vi "Show One Plot.vi"() -> ()   [LabVIEW 2012]
uses:
  <vilib>/Utility/miscctls.llb/LVRangeTypeDef.ctl
  <vilib>/Utility/miscctls.llb/LVPointDoubleTypeDef.ctl
  Type/_Data Operation.ctl
  <vilib>/printing/EasyPrintingControls.llb/layout_options.ctl
  <vilib>/printing/EasyPrintingControls.llb/orientation.ctl
  <vilib>/printing/EasyPrintingControls.llb/panel_scaling_for_page.ctl
  <vilib>/printing/EasyPrintingControls.llb/margins.ctl
  <vilib>/printing/EasyPrintingControls.llb/margin_values.ctl
  <vilib>/printing/EasyPrintingControls.llb/measurement_system.ctl
  <vilib>/printing/EasyPrintingControls.llb/printer_options.ctl
  <vilib>/printing/EasyPrintingControls.llb/printing_method.ctl
  <vilib>/printing/EasyPrintingControls.llb/color_or_monochrome.ctl
  <vilib>/printing/EasyPrintingControls.llb/page_header_options.ctl
  <vilib>/printing/EasyPrintingControls.llb/page_headers.ctl
  <vilib>/printing/EasyPrintingControls.llb/page_header_content_options.ctl
  <vilib>/printing/EasyPrinting.llb/Easy Print VI Panel or Documentation (path).vi
  <vilib>/Utility/NIReport.llb/NI_ReportGenerationCore.lvlib
panel:
  in  "Data":T3
  in  "Expt#":i32=1 caption="Experiment #"
  out "Scan #":i32=1
  out "Run Time":i32=1 caption="Run Time (ms)"
  out "Plot":cluster{"TIC X":dbl[], "TIC Y":dbl[]}[](graph)
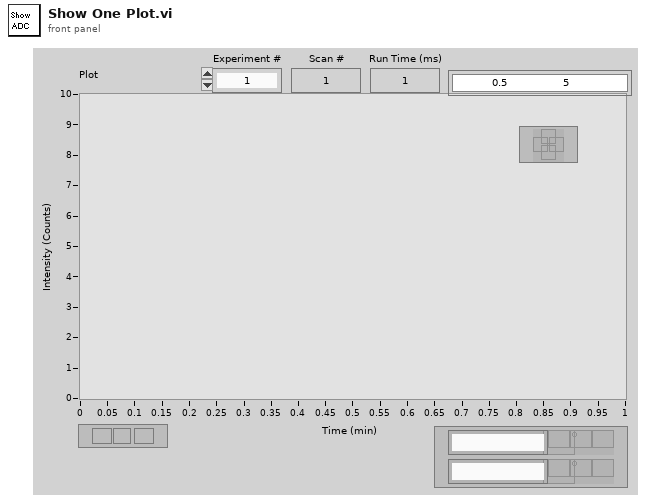
[diagram p1: front panel]
types:
  T1 = typedef "LVRangeTypeDef.ctl" = cluster{"Minimum":dbl, "Maximum":dbl, "Increment":dbl, "Minor Increment":dbl, "Start":dbl}
  T2 = typedef "LVPointDoubleTypeDef.ctl" = cluster{"X":dbl, "Y":dbl}
  T3 = cluster{"YScale.NameLbl.Text":string, "XScale.NameLbl.Text":string, "XScale.Range":T1, "YScale.Range":T1, "Label.Text":string, "Cursor.Cursor Position":T2, "Plot.Bar Plot Style":u8}
  T4 = typedef "_Data Operation.ctl" = enum8{"Initialize", "Get Data", "Set Data", "Close"}
  T5 = typedef "NI_ReportGenerationCore.lvlib/layout_options.ctl" = cluster{"orientation (unchanged)":T6, "panel scaling for page (unchanged)":T7, "margins":T8, "printer options":T11, "page header options":T14}
  T6 = typedef "NI_ReportGenerationCore.lvlib/orientation.ctl" = u16
  T7 = typedef "NI_ReportGenerationCore.lvlib/panel_scaling_for_page.ctl" = u16
  T8 = typedef "NI_ReportGenerationCore.lvlib/margins.ctl" = cluster{"override VI margins (false)":bool, "margins (1.00)":T9, "measurement system (default)":T10}
  T9 = typedef "NI_ReportGenerationCore.lvlib/margin_values.ctl" = cluster{"top":dbl, "left":dbl, "right":dbl, "bottom":dbl}
  T10 = typedef "NI_ReportGenerationCore.lvlib/measurement_system.ctl" = u16
  T11 = typedef "NI_ReportGenerationCore.lvlib/printer_options.ctl" = cluster{"destination printer name (current)":string, "printing method (unchanged)":T12, "color or monochrome (unchanged)":T13}
  T12 = typedef "NI_ReportGenerationCore.lvlib/printing_method.ctl" = u16
  T13 = typedef "NI_ReportGenerationCore.lvlib/color_or_monochrome.ctl" = u16
  T14 = typedef "NI_ReportGenerationCore.lvlib/page_header_options.ctl" = cluster{"page headers (unchanged)":T15, "page header content options":T16}
  T15 = typedef "NI_ReportGenerationCore.lvlib/page_headers.ctl" = u16
  T16 = typedef "NI_ReportGenerationCore.lvlib/page_header_content_options.ctl" = cluster{"Include VI Name":bool, "Include VI Path":bool, "Include Last Modification Date":bool, "Include Date Printed":bool, "Include Page Number":bool, "Include VI Icon":bool}
  T17 = typedef "_Current Data.ctl" = cluster{"Scan#":i32, "Run Time (mS)":i32, "TIC X":dbl[], "TIC Y":dbl[][], "MassRange":cluster{"X Title":string, "X":dbl[], "Y":i32[]}[], "Fixed Mass (amu)":dbl, "Method":T18}
  T18 = typedef "_XML Expt.ctl" = cluster{"StartT(mS)":i32, "#Cycles":i32, "PauseT(uS)":i32, "ScanType":i32, "Polarity":u8, "FixedMass":dbl, "DelayT(mS)":i32, "Active Ch":T19[], "Mass Range":T20[]}
  T19 = typedef "_XML Lens.ctl" = cluster{"Value":dbl, "ChID":u8}
  T20 = typedef "_Mass Range Property.ctl" = cluster{"Start":dbl, "Stop":dbl, "Step Size":dbl, "Steps":i32, "Dwell":dbl, "Parameters":T21[], "Res":T22}
  T21 = typedef "_Mass Range Parameters.ctl" = cluster{"Name":string, "Ch#":u8, "StartV":dbl, "StopV":dbl, "StepV":dbl, "Index":u8}
  T22 = typedef "_RT Res Type.ctl" = u16
  T23 = cluster{"Data":cluster{"X":dbl[], "Y":dbl[]}, "Y Title":string, "X Title":string}
  T24 = typedef "imagedata.ctl" = cluster{"image type":i32, "image depth":i32, "image":u8[], "mask":u8[], "colors":u32[], "Rectangle":cluster{"left":i16, "top":i16, "right":i16, "bottom":i16}}
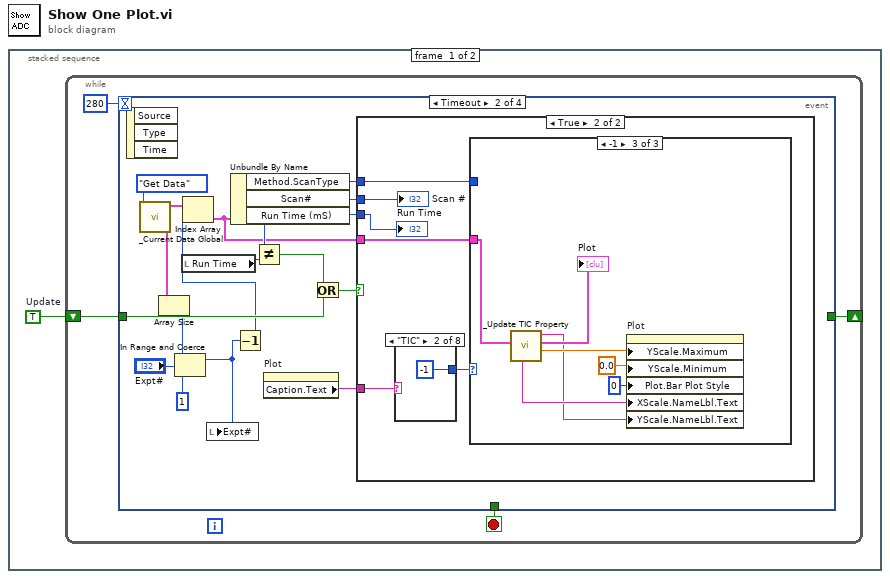
[diagram p0: block diagram]
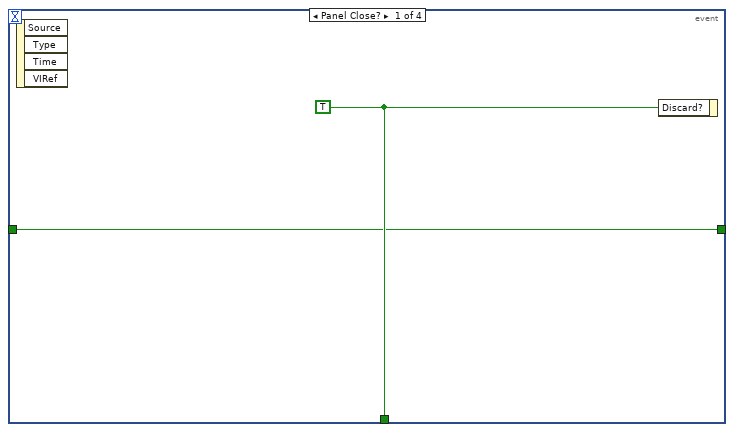
[diagram p2: hidden frame]
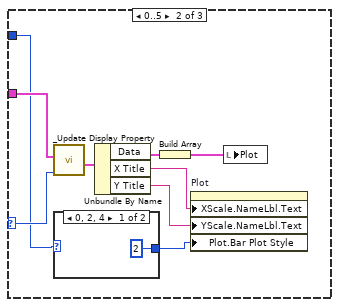
[diagram p5: hidden frame]
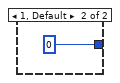
[diagram p6: hidden frame]
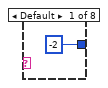
[diagram p7: hidden frame]
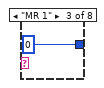
[diagram p8: hidden frame]
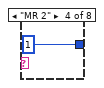
[diagram p9: hidden frame]
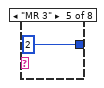
[diagram p10: hidden frame]
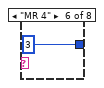
[diagram p11: hidden frame]
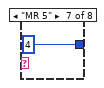
[diagram p12: hidden frame]
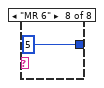
[diagram p13: hidden frame]
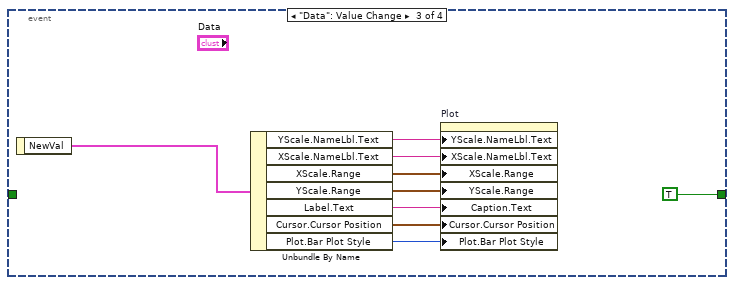
[diagram p14: hidden frame]
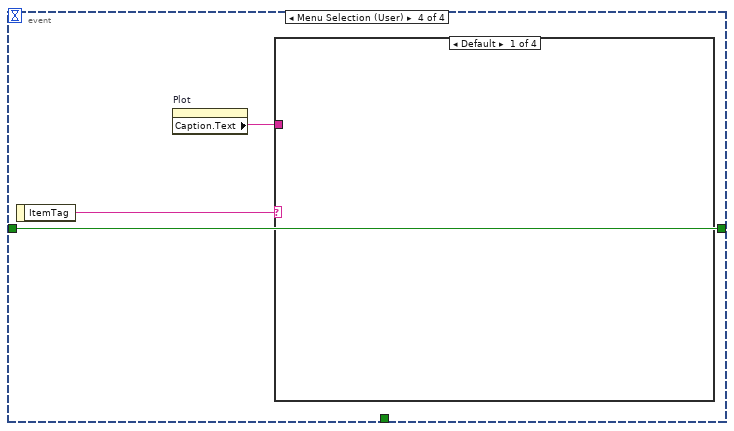
[diagram p15: hidden frame]
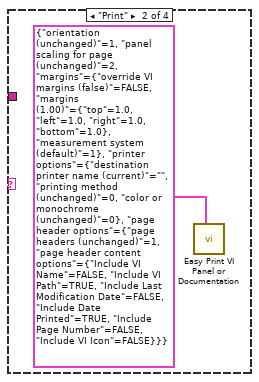
[diagram p16: hidden frame]
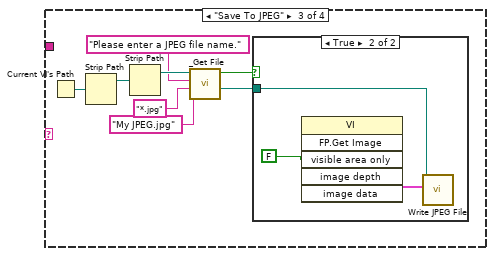
[diagram p17: hidden frame]
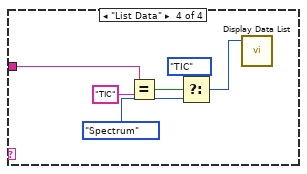
[diagram p19: hidden frame]
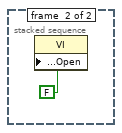
[diagram p20: hidden frame]
diagram:
  n1 = stacked-sequence {
    frame #0 {
      w1 = TRUE  # Update
      n2 = while {
        shift-right: [w2] -> _
        shift-left: w1 -> [w3]
        stop <- w5 stop-if-true
        n3 = event shown="[1] Timeout" {
          selector: _ -> [_ _ _ _]
          dyn-events: _ -> [_ _ _ _]
          timeout: 280 -> [_ _ _ _]
          tunnel: [w7 _ _ _] -> w5
          tunnel: w3 -> [w6 w22 _ w65]
          tunnel: [w6 _ TRUE ("Update") w65] -> w2
          event Panel Close? {
            w7 = TRUE ("Discard?")
            n4 = event-data() -> ()  [unwired: 5 out]
            n5 = event-data("Discard?"=w7) -> ()  [unwired: 1 in, 1 out]
          }
          event Timeout {
            n6 = event-data() -> ()  [unwired: 4 out]
            n7 = call "_Current Data Global.vi"("Operation"=_Data_Operation."Get Data") -> ("CurrentData"=w13:T17[])  [unwired: 3 in, 3 out]
            n8 = Array Size(array=w13) -> (size(s)=w14:i32)
            n9 = In Range and Coerce(upper limit=w14, x="Expt#", lower limit=1) -> (coerced(x)=w10:i32)  [unwired: 1 out]
            n10 = local read "Run Time"() -> (w18:i32)
            n11 = local write "Expt#"(w10) -> ()
            n12 = Decrement(x=w10) -> (x-1=w9:i32)
            n13 = Index Array(array=w13, index=w9) -> (element=w15:T17)
            n14 = Unbundle By Name(w15) -> ("Method.ScanType"=w8:i32, "Scan#"=w19:i32, "Run Time (mS)"=w17:i32)
            n15 = Not Equal?(x=w17, y=w18) -> (x != y?=w16:bool)
            n16 = property on="Plot" class="XYGraph (strict)"() -> ("Caption.Text"=w23:string)  [unwired: 2 in, 2 out]
            n17 = Or(x=w16, y=w22) -> (x .or. y?=w21:bool)
            n18 = case shown="True" w21 {
              tunnel: w23 -> [_ w29]
              tunnel: w17 -> [_ w26]
              tunnel: w19 -> [_ w27]
              tunnel: w15 -> [_ w25]
              tunnel: w8 -> [_ w24]
              frame False {
              }
              frame True {
                n19 = case shown="\"TIC\"" w29 {
                  tunnel: [-2 -1 0 1 2 3 4 5] -> w28
                  frame Default {
                  }
                  frame "TIC" {
                  }
                  frame "MR 1" {
                  }
                  frame "MR 2" {
                  }
                  frame "MR 3" {
                  }
                  frame "MR 4" {
                  }
                  frame "MR 5" {
                  }
                  frame "MR 6" {
                  }
                }
                n20 = case shown="-1" w28 {
                  selector: w28 -> [_ w38 _]
                  tunnel: w25 -> [_ w32 w45]
                  tunnel: w24 -> [_ w31 _]
                  frame Default {
                  }
                  frame 0..5 {
                    n21 = call "_Update Display Property.vi"("MassRange# (0)"=w38, "Current Data"=w32) -> ("Graph Data"=w37:T23)  [unwired: 2 in, 4 out]
                    n22 = case shown="0, 2, 4" w31 {
                      tunnel: [u8 2 ("Plot.Bar Plot Style") u8 0 ("Plot.Bar Plot Style")] -> w30
                      frame 0, 2, 4 {
                      }
                      frame 1, Default {
                      }
                    }
                    n23 = Unbundle By Name(w37) -> ("Data"=w36:cluster{"X":dbl[], "Y":dbl[]}, "X Title"=w34:string, "Y Title"=w33:string)
                    n24 = Build Array(w36) -> (w35:cluster{"X":dbl[], "Y":dbl[]}[])
                    n25 = property on="Plot" class="XYGraph (strict)"("XScale.NameLbl.Text"=w34, "YScale.NameLbl.Text"=w33, "Plot.Bar Plot Style"=w30) -> ()  [unwired: 2 in, 2 out]
                    n26 = local write "Plot"(w35) -> ()
                  }
                  frame -1 {
                    n27 = call "_Update TIC Property.vi"("Current Data"=w45) -> ("YMax"=w43:dbl, "TIC Data"=→"Plot":cluster{"TIC X":dbl[], "Data in cps":dbl[]}[], "YTitle"=w41:string, "XTitle"=w42:string)  [unwired: 7 out]
                    n28 = property on="Plot" class="XYGraph (strict)"("YScale.Maximum"=w43, "YScale.Minimum"=0.0 ("Y Scale.Range:Minimum"), "Plot.Bar Plot Style"=u8 0, "XScale.NameLbl.Text"=w42, "YScale.NameLbl.Text"=w41) -> ()  [unwired: 2 in, 2 out]
                  }
                }
                "Scan #" <- w27
                "Run Time" <- w26
              }
            }
          }
          event "Data": Value Change {
            n29 = event-data() -> ("NewVal"=w63:T3)  [unwired: 1 out]
            n30 = Unbundle By Name(w63) -> ("YScale.NameLbl.Text"=w57:string, "XScale.NameLbl.Text"=w58:string, "XScale.Range"=w59:T1, "YScale.Range"=w60:T1, "Label.Text"=w61:string, "Cursor.Cursor Position"=w62:T2, "Plot.Bar Plot Style"=w56:u8)
            n31 = property on="Plot" class="XYGraph (strict)"("YScale.NameLbl.Text"=w57, "XScale.NameLbl.Text"=w58, "XScale.Range"=w59, "YScale.Range"=w60, "Caption.Text"=w61, "Cursor.Cursor Position"=w62, "Plot.Bar Plot Style"=w56) -> ()  [unwired: 2 in, 2 out]
          }
          event Menu Selection (User) {
            n32 = event-data() -> ("ItemTag"=w67:string)  [unwired: 1 out]
            n33 = property on="Plot" class="XYGraph (strict)"() -> ("Caption.Text"=w66:string)  [unwired: 2 in, 2 out]
            n34 = case shown="Default" w67 {
              tunnel: w66 -> [_ _ _ w80]
              frame Default {
              }
              frame "Print" {
                n35 = call-poly <vilib>:"Easy Print VI Panel or Documentation.vi"("layout options"=T5 {"orientation (unchanged)"=1, "panel scaling for page (unchanged)"=2, "margins"={"override VI margins (false)"=FALSE, "margins (1.00)"={"top"=1.0, "left"=1.0, "right"=1.0, "bottom"=1.0}, "measurement system (default)"=1}, "printer options"={"destination printer name (current)"="", "printing method (unchanged)"=0, "color or monochrome (unchanged)"=0}, "page header options"={"page headers (unchanged)"=1, "page header content options"={"Include VI Name"=FALSE, "Include VI Path"=TRUE, "Include Last Modification Date"=FALSE, "Include Date Printed"=TRUE, "Include Page Number"=FALSE, "Include VI Icon"=FALSE}}}) -> ()  [unwired: 4 in, 7 out]
              }
              frame "Save To JPEG" {
                n36 = Current VI's Path() -> (path=w76:path)
                n37 = Strip Path(path=w76) -> (stripped path=w75:path)  [unwired: 1 out]
                n38 = Strip Path(path=w75) -> (stripped path=w74:path)  [unwired: 1 out]
                n39 = call "_Get File.vi"("default name"="My JPEG.jpg", "extension (isd)"="*.jpg", "prompt"="Please enter a JPEG file name.", "Start Path"=w74) -> ("Seleted File"=w69:path, "Succeeded"=w70:bool)  [unwired: 2 in, 2 out]
                n40 = case shown="True" w70 {
                  tunnel: w69 -> [_ w77]
                  frame False {
                  }
                  frame True {
                    n41 = invoke class="VI" method="FP.Get Image"("visible area only"=FALSE ("Visible Area Only")) -> ("image data"=w78:T24)  [unwired: 5 in, 5 out]
                    n42 = call <vilib>:"Write JPEG File.vi"("image data"=w78, "path to JPEG file"=w77) -> ()  [unwired: 1 in, 9 out]
                  }
                }
              }
              frame "List Data" {
                n43 = Equal?(x=w80, y="TIC") -> (x = y?=w84:bool)
                n44 = Select(t=enum16{"TIC", "Spectrum", "Peak"}."TIC" ("Data Type"), s=w84, f=enum16{"TIC", "Spectrum", "Peak"}."Spectrum" ("Data Type")) -> (s? t:f=w81:enum16{"TIC", "Spectrum", "Peak"})
                n45 = call "Display Data List.vi"("Data Type"=w81) -> ()  [unwired: 3 in, 6 out]
              }
            }
          }
        }
      }
    }
    frame #1 {
      n46 = property class="VI"("Front Panel.Open"=FALSE ("Front Panel Window:Open")) -> ()  [unwired: 2 in, 2 out]
    }
  }
